vi "Write Module Name.vi"(8 "error in (no error)":errorcluster, 10 "Module Name":string, 11 "Rename in":refnum<class "Rename.lvclass">) -> (0 "error out":errorcluster, 3 "Rename out":refnum<class "Rename.lvclass">)   [LabVIEW 2015, in "Generic Module Library.lvlib" / "Template G_Module.lvlib" / "Rename.lvclass"]
uses:
  Rename.lvclass
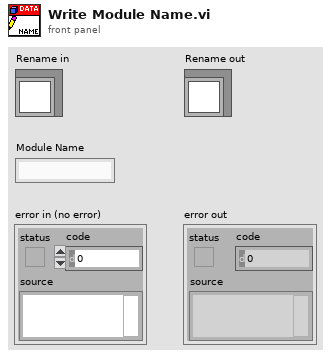
[diagram p1: front panel]
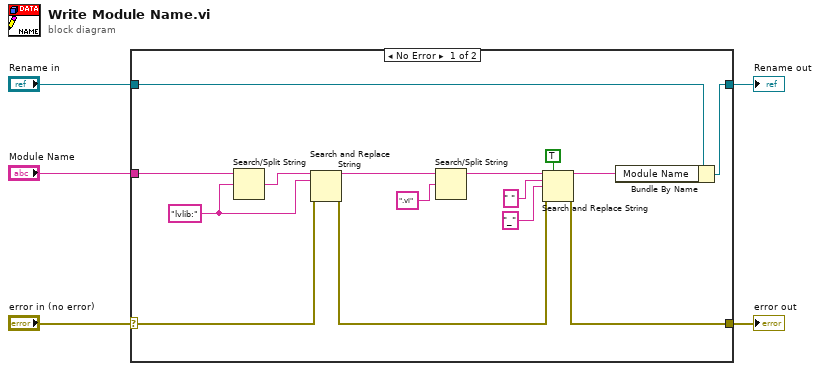
[diagram p0: block diagram]
diagram:
  n1 = case shown="No Error" "error in (no error)" {
    selector: "error in (no error)" -> [w8 w21]
    tunnel: [w15 w21] -> w4
    tunnel: [w19 w22] -> w2
    tunnel: "Rename in" -> [w20 w22]
    tunnel: "Module Name" -> [w13 _]
    frame No Error {
      w9 = "lvlib:" ("search string/char (-)")
      n2 = Search/Split String(string=w13, search string/char (-)=w9) -> (match + rest of string=w6:string)  [unwired: 1 in, 2 out]
      n3 = Search and Replace String(input string=w6, search string=w9, error in=w8) -> (result string=w10:string, error out=w7:errorcluster)  [unwired: 5 in, 2 out]
      n4 = Search/Split String(string=w10, search string/char (-)=".vi") -> (substring before match=w11:string)  [unwired: 1 in, 2 out]
      n5 = Search and Replace String(replace all?=TRUE ("replace all? (F)"), input string=w11, search string=" ", replace string="_" ("replace string (\"\")"), error in=w7) -> (result string=w14:string, error out=w15:errorcluster)  [unwired: 3 in, 2 out]
      n6 = Bundle By Name(cluster=w20, "Module Name"=w14) -> (w19:refnum<class "Rename.lvclass">)
    }
    frame Error {
    }
  }
  "error out" <- w4
  "Rename out" <- w2
